vi "Measurement.Free.GetConfiguration.vi"(8 "error in (no error)":errorcluster, 11 "Measurement.Free":refnum<class "Measurement.Free.lvclass">) -> (0 "error out":errorcluster, 2 "Configuration":T1, 3 "Measurement.Free out":refnum<class "Measurement.Free.lvclass">)   [LabVIEW 2017, in "Measurement.Free.lvclass"]
doc: "---------------------------------------------------------------\nJKI State Machine Objects™\nhttp://jki.net/state-machine-objects/\nCopyright (C) 2005-2015, JKI <info@jki.net>\nALL RIGHTS RESERVEDJKI State Machine Objects (SMO) 1.0.0.5\nJKI - JKI\nCopyright (c) 2016, JKI"
uses:
  Measurement.Free.lvclass
  Typedefs/Configuration--Cluster.ctl
  Typedefs/Configuration.Hardware--Cluster.ctl
  Typedefs/Configuration.SMU--Cluster.ctl
  SMU/Typedefs/Configuration--Cluster.ctl
  Typedefs/Configuration.LIA--Cluster.ctl
  LIA/Typedefs/Configuration--Cluster.ctl
  Typedefs/Configuration.OPM--Cluster.ctl
  OPM/Typedefs/Configuration--Cluster.ctl
  Typedefs/Configuration.OPA--Cluster.ctl
  OPA/Typedefs/Configuration--Cluster.ctl
  Measurement.Free.lvclass/Measurement.Free.ctl
  SMU/SMU.lvclass
  LIA/LIA.lvclass
  OPM/OPM.lvclass
  OPA/OPA.lvclass
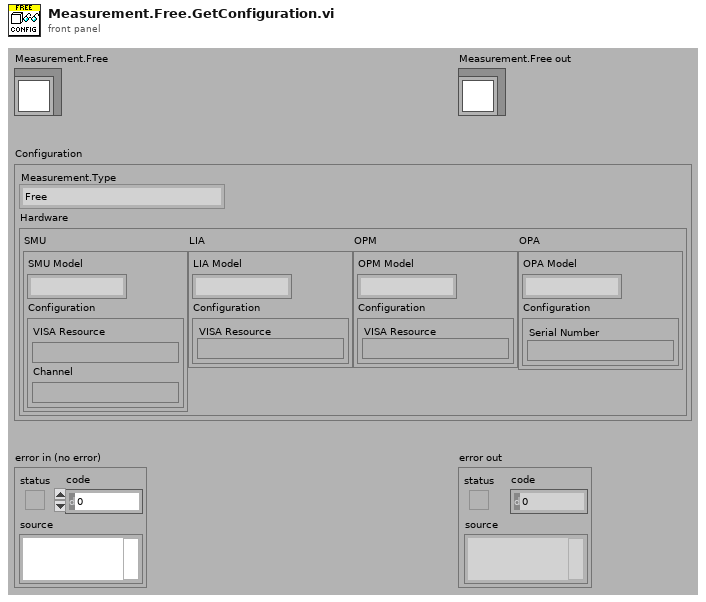
[diagram p1: front panel]
types:
  T1 = typedef "Measurement.Free.lvclass/Configuration--Cluster.ctl" = cluster{"Measurement.Type":enum16{"Free", "I/V Curve", "Wavelength sweeping", "Photocurrent mapping"}, "Hardware":T2}
  T2 = typedef "Measurement.Free.lvclass/Configuration.Hardware--Cluster.ctl" = cluster{"SMU":T3, "LIA":T5, "OPM":T7, "OPA":T9}
  T3 = typedef "Measurement.Free.lvclass/Configuration.SMU--Cluster.ctl" = cluster{"SMU Model":string, "Configuration":T4}
  T4 = typedef "SMU.lvclass/Configuration--Cluster.ctl" = cluster{"VISA Resource":string, "Channel":string}
  T5 = typedef "Measurement.Free.lvclass/Configuration.LIA--Cluster.ctl" = cluster{"LIA Model":string, "Configuration":T6}
  T6 = typedef "LIA.lvclass/Configuration--Cluster.ctl" = cluster{"VISA Resource":string}
  T7 = typedef "Measurement.Free.lvclass/Configuration.OPM--Cluster.ctl" = cluster{"OPM Model":string, "Configuration":T8}
  T8 = typedef "OPM.lvclass/Configuration--Cluster.ctl" = cluster{"VISA Resource":string}
  T9 = typedef "Measurement.Free.lvclass/Configuration.OPA--Cluster.ctl" = cluster{"OPA Model":string, "Configuration":T10}
  T10 = typedef "OPA.lvclass/Configuration--Cluster.ctl" = cluster{"Serial Number":string}
  T11 = typedef "Measurement.Free.lvclass/PrivateData--Ref.ctl" = refnum<data-value>
  T12 = typedef "Measurement.Free.lvclass/PrivateData--Cluster.ctl" = cluster{"Configuration":T1, "Public Events":T13, "Protected Events":T14, "Private Events":T15, "Data":T16}
  T13 = typedef "Measurement.Free.lvclass/PublicEvents--Cluster.ctl" = cluster{"Data Changed":refnum<user-event>}
  T14 = typedef "Measurement.Free.lvclass/ProtectedEvents--Cluster.ctl" = cluster{"API_Template":refnum<user-event>}
  T15 = typedef "Measurement.Free.lvclass/PrivateEvents--Cluster.ctl" = cluster{"Initialize":refnum<user-event>}
  T16 = typedef "Measurement.Free.lvclass/Data.ctl" = string
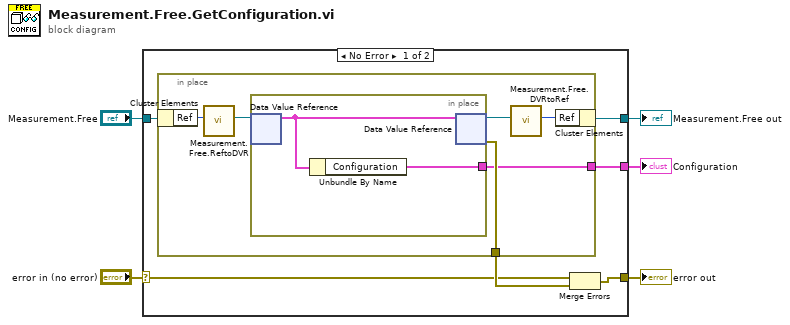
[diagram p0: block diagram]
diagram:
  n1 = case shown="No Error" "error in (no error)" {
    selector: "error in (no error)" -> [w7 w20]
    tunnel: "Measurement.Free" -> [w8 w21]
    tunnel: [w9 w20] -> w4
    tunnel: [w11 w21] -> w3
    tunnel: [w6 _] -> w1
    frame No Error {
      n2 = in-place {
        in-place-border: [w17] -> w10
        in-place-border: [w12] -> w6
        n3 = in-place-cluster #1(w8) -> ("Ref"=w16:u32)
        n4 = call "Measurement.Free.ReftoDVR.vi"("Ref"=w16) -> ("Ref"=w15:T11)  [unwired: 10 in]
        n5 = in-place {
          in-place-border: [w18] -> w12
          n6 = in-place-dvr #2(w15) -> (w19:T12)  [unwired: 1 out]
          n7 = Unbundle By Name(w19) -> ("Configuration"=w18:T1)
          n8 = in-place-dvr #2(w19) -> (w14:T11, w17:errorcluster)
        }
        n9 = call "Measurement.Free.DVRtoRef.vi"("Ref"=w14) -> ("Ref"=w13:u32)  [unwired: 10 in]
        n10 = in-place-cluster #1("Ref"=w13) -> (w11:refnum<class "Measurement.Free.lvclass">)
      }
      n11 = Merge Errors(w7, w10) -> (w9:errorcluster)
    }
    frame Error {
    }
  }
  "error out" <- w4
  "Measurement.Free out" <- w3
  "Configuration" <- w1
